vi "BufferArray.vi"(9 "Index":i32, 10 "Total amount of Pts":i32, 11 "Input Y-values":dbl[](array[numeric])) -> (3 "Output Array":dbl[](array[numeric]))   [LabVIEW 2014]
panel:
  # "BufferArray.VI"
  # "Inputs"
  # "Outputs"
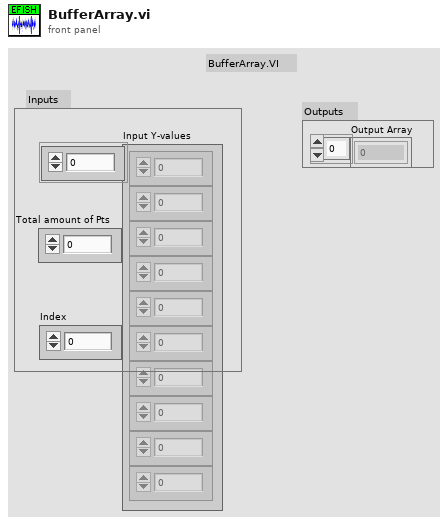
[diagram p1: front panel]
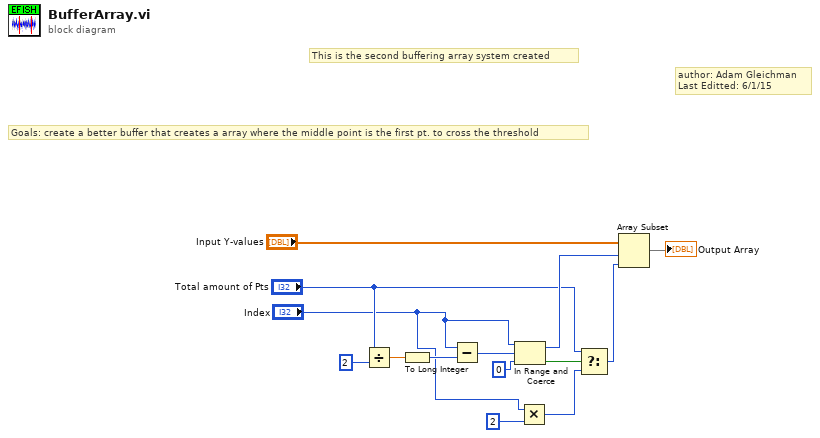
[diagram p0: block diagram]
diagram:
  # "author: Adam Gleichman\nLast Editted: 6/1/15"
  # "This is the second buffering array system created"
  # "Goals: create a better buffer that creates a array where the middle point is the first pt. to cross the threshold"
  n1 = Divide(x="Total amount of Pts", y=2) -> (x/y=w12:dbl)
  n2 = To Long Integer(number=w12) -> (32bit integer=w8:i32)
  n3 = Subtract(x="Index", y=w8) -> (x-y=w7:i32)
  n4 = In Range and Coerce(upper limit="Index", x=w7, lower limit=0) -> (coerced(x)=w10:i32, In Range?=w6:bool)
  n5 = Multiply(x="Index", y=2) -> (x*y=w4:i32)
  n6 = Select(t="Total amount of Pts", s=w6, f=w4) -> (s? t:f=w2:i32)
  n7 = Array Subset(array="Input Y-values", index=w10, length=w2) -> (→"Output Array":dbl[])
